vi "Intake.vi"() -> ()   [LabVIEW 2013]
uses:
  Globals/Homes.vi
  Globals/Useful Values.vi
  <vilib>/Rock Robotics/WPI/Joystick/WPI_JoystickGetSetRefNum.vi
  Robot Global Data.vi
  Globals/Auto.vi
  <vilib>/addons/control/pid/pid.llb/PID (DBL).vi
  <vilib>/addons/control/pid/NI_PID_pid.lvlib
panel:
  in  "x":dbl format="%#_13g"
  in  "PID gains Ultrasonic":T1={"proportional gain (Kc)"=12.0, "integral time (Ti, min)"=0.0, "derivative time (Td, min)"=0.0} {"derivative time (Td, min)" format="%.3f"; "integral time (Ti, min)" format="%.3f"; "proportional gain (Kc)" format="%.3f"}
  in  "Ultrasonic":dbl=0.6
  in  "Negate?":bool=TRUE
  out "Motor Output":dbl
  out "Intake Voltage":dbl=0.7652226560000001
  in  "PID gains":T1={"proportional gain (Kc)"=3.6, "integral time (Ti, min)"=0.0, "derivative time (Td, min)"=0.0} {"derivative time (Td, min)" format="%.3f"; "integral time (Ti, min)" format="%.3f"; "proportional gain (Kc)" format="%.3f"}
  out "Setpoint":dbl=0.75
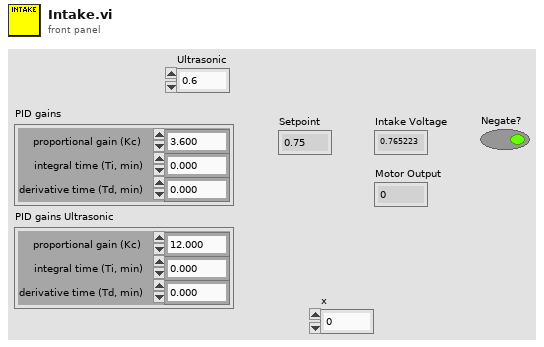
[diagram p1: front panel]
types:
  T1 = cluster{"proportional gain (Kc)":dbl, "integral time (Ti, min)":dbl, "derivative time (Td, min)":dbl}
  T2 = typedef "WPI_MotorControlDeviceRef.ctl" = cluster{"DeviceStatus":errorcluster, "Type":enum16{"PWM", "CAN"}, "PWM":cluster{"Digital Module":T3, "PWM Channel":T4, "DeadBand":T5}, "CAN":cluster{"Device Number":u8, "Control Mode":T6, "Semaphore":T7, "Max Vout":dbl}, "Invert":bool, "TransformRef":T8, "InvTransformRef":T8}
  T3 = typedef "FPGA_TypedefDigitalModule.ctl" = enum16{"Digital Module 1", "Digital Module 2"}
  T4 = typedef "FPGA_DIOPWMChannel.ctl" = enum8{"PWM 1", "PWM 2", "PWM 3", "PWM 4", "PWM 5", "PWM 6", "PWM 7", "PWM 8", "PWM 9", "PWM 10", "Invalid"}
  T5 = typedef "WPI_PWMDeadband.ctl" = cluster{"Name":string, "maxPositivePwm":i32, "minPositivePwm":i32, "centerPwm":i32, "maxNegativePwm":i32, "minNegativePwm":i32, "angularRange":u16}
  T6 = typedef "WPI_CANJaguar_ControlMode.ctl" = enum8{"Percent VBus", "Current", "Speed", "Position", "Voltage"}
  T7 = typedef "Semaphore RefNum" = refnum<k1>
  T8 = typedef "WPI_PWMTransform_ConPane.ctl" = refnum<vi>
  T9 = typedef "WPI_JoystickDevRef.ctl" = cluster{"Device":T10}
  T10 = typedef "WPI_JoystickDeviceEnum.ctl" = enum16{"USB 1", "USB 2", "USB 3", "USB 4", "Kinect 1", "Kinect 2"}
  T11 = typedef "WPI_AnalogChannelDevRef.ctl" = cluster{"DevStatus":errorcluster, "Analog Module":T12, "Analog Channel":T13}
  T12 = typedef "FPGA_TypedefAnalogModule.ctl" = enum16{"Analog Module 1", "Analog Module 2"}
  T13 = typedef "FPGA_AIChannel.ctl" = enum8{"AI 1", "AI 2", "AI 3", "AI 4", "AI 5", "AI 6", "AI 7", "AI 8", "Invalid"}
  T14 = typedef "WPI_DriverStationRobotMode2.ctl" = enum16{"Autonomous Disabled", "Autonomous Enabled", "Teleop Disabled", "Teleop Enabled", "Timeout", "Finish", "Test Disabled", "Test Enabled"}
  T15 = typedef "WPI_JoystickButtonState.ctl" = cluster{"Button 1":bool, "Button 2":bool, "Button 3":bool, "Button 4":bool, "Button 5":bool, "Button 6":bool, "Button 7":bool, "Button 8":bool, "Button 9":bool, "Button 10":bool, "Button 11":bool, "Button 12":bool}
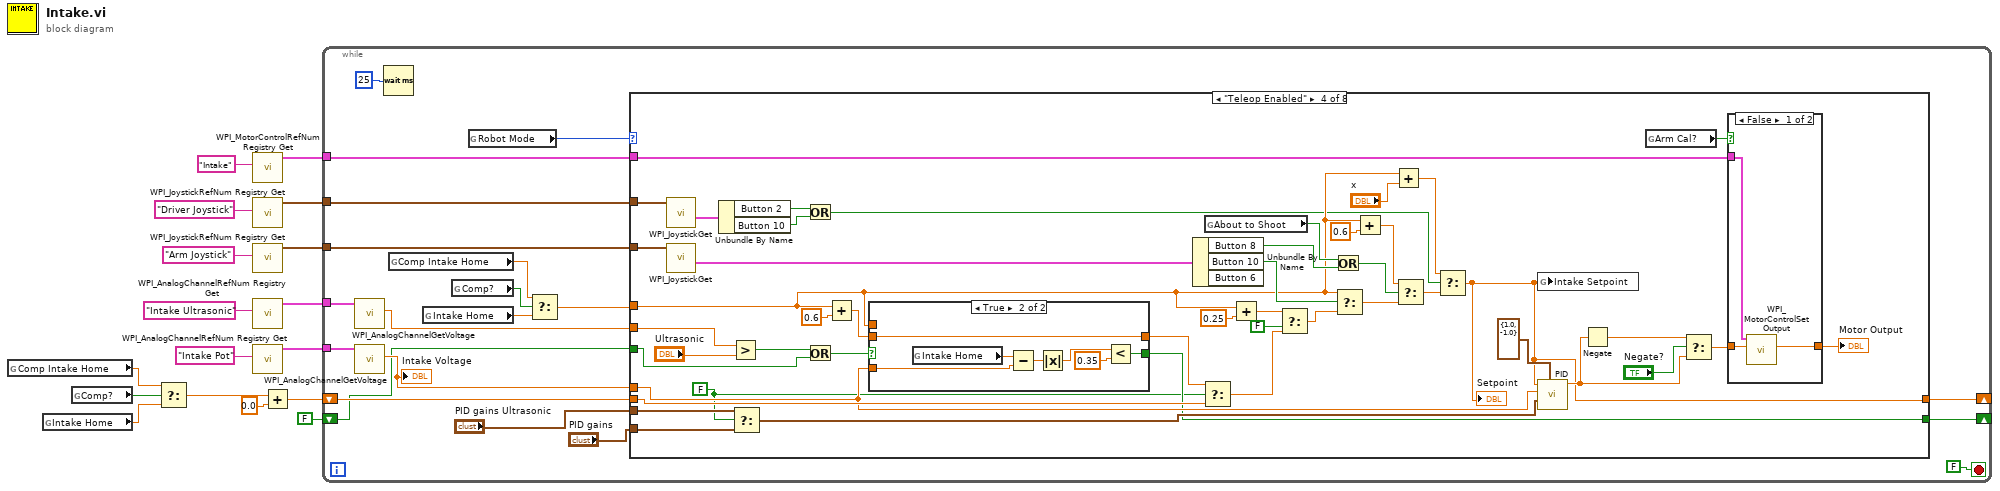
[diagram p0: block diagram]
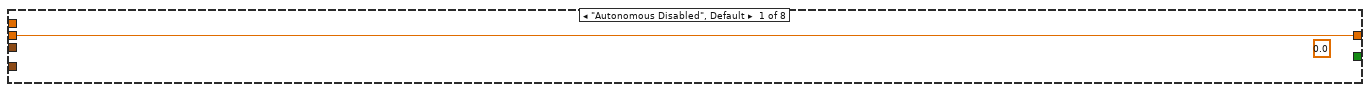
[diagram p2: hidden frame]
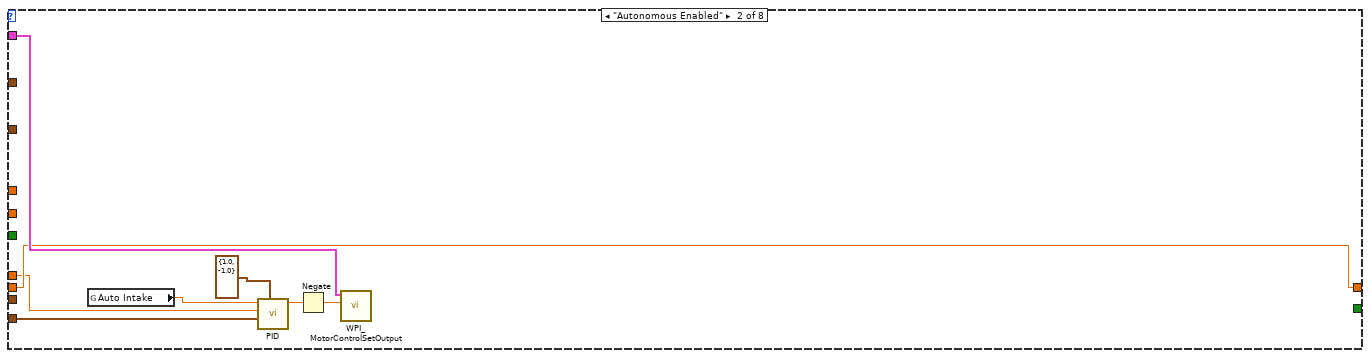
[diagram p3: hidden frame]
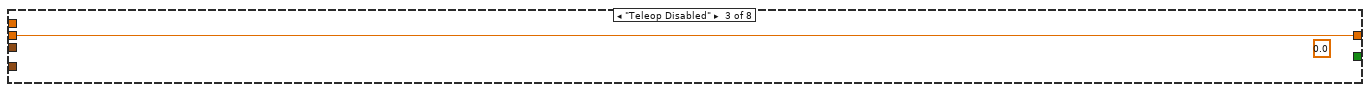
[diagram p4: hidden frame]
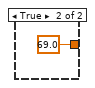
[diagram p5: hidden frame]
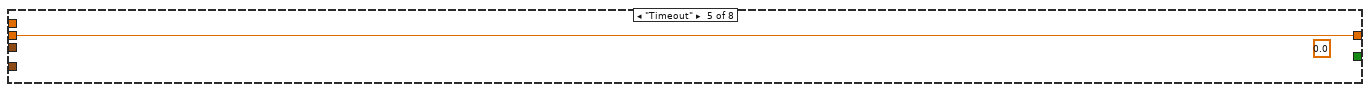
[diagram p7: hidden frame]
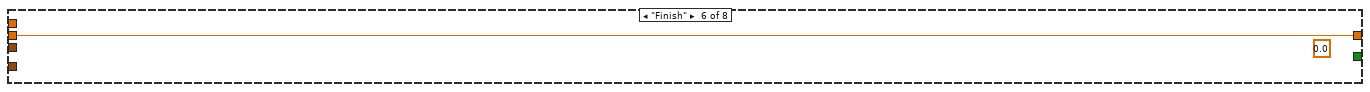
[diagram p8: hidden frame]
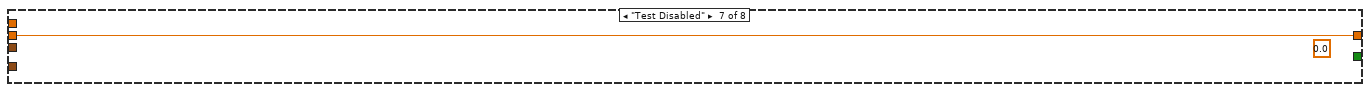
[diagram p9: hidden frame]
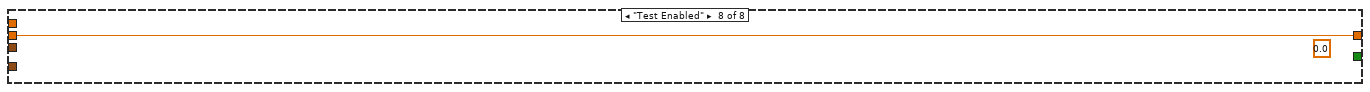
[diagram p10: hidden frame]
diagram:
  n1 = global read "Homes.vi" "Comp Intake Home"() -> (w9:dbl)
  n2 = global read "Homes.vi" "Intake Home"() -> (w10:dbl)
  n3 = global read "Useful Values.vi" "Comp?"() -> (w11:bool)
  n4 = Select(t=w9, s=w11, f=w10) -> (s? t:f=w8:dbl)
  n5 = call <vilib>:"WPI_MotorControlRefNum Registry Get.vi"("refnum name"="Intake") -> ("MotorControlDevRef"=w14:T2)  [unwired: 9 in, 1 out]
  n6 = call <vilib>:"WPI_JoystickRefNum Registry Get.vi"("refnum name"="Driver Joystick") -> ("JoystickDevRef"=w1:T9)  [unwired: 9 in, 1 out]
  n7 = call <vilib>:"WPI_JoystickRefNum Registry Get.vi"("refnum name"="Arm Joystick") -> ("JoystickDevRef"=w12:T9)  [unwired: 9 in, 1 out]
  n8 = call <vilib>:"WPI_AnalogChannelRefNum Registry Get.vi"("refnum name"="Intake Ultrasonic") -> ("AIDeviceRef"=w4:T11)  [unwired: 9 in, 1 out]
  n9 = call <vilib>:"WPI_AnalogChannelRefNum Registry Get.vi"("refnum name"="Intake Pot") -> ("AIDeviceRef"=w17:T11)  [unwired: 9 in, 1 out]
  n10 = Add(x=w8, y=0.0 ("x")) -> (x+y=w7:dbl)
  n11 = while {
    tunnel: w17 -> [w35]
    tunnel: w14 -> [w33]
    tunnel: w12 -> [w30]
    shift-right: [w28] -> _
    shift-left: w7 -> [w29]
    tunnel: w4 -> [w23]
    shift-right: [w20] -> _
    shift-left: FALSE -> [w19]
    tunnel: w1 -> [w18]
    stop <- FALSE stop-if-true
    n12 = call <vilib>:"WPI_AnalogChannelGetVoltage.vi"("AIDeviceRef"=w23) -> ("Voltage"=w22:dbl)  [unwired: 8 in, 2 out]
    n13 = call <vilib>:"WPI_AnalogChannelGetVoltage.vi"("AIDeviceRef"=w35) -> ("Voltage"=w32:dbl)  [unwired: 8 in, 2 out]
    "Intake Voltage" <- w32
    n14 = Wait (ms)(milliseconds to wait=u32 25) -> ()  [unwired: 1 out]
    n15 = global read "Homes.vi" "Comp Intake Home"() -> (w27:dbl)
    n16 = global read "Homes.vi" "Intake Home"() -> (w26:dbl)
    n17 = global read "Useful Values.vi" "Comp?"() -> (w25:bool)
    n18 = global read "Robot Global Data.vi" "Robot Mode"() -> (w34:T14)
    n19 = Select(t=w27, s=w25, f=w26) -> (s? t:f=w24:dbl)
    n20 = case shown="\"Teleop Enabled\"" w34 {
      tunnel: w33 -> [_ w44 _ w52 _ _ _ _]
      tunnel: w32 -> [_ w42 _ w70 _ _ _ _]
      tunnel: "PID gains" -> [_ w45 _ w73 _ _ _ _]
      tunnel: w30 -> [_ _ _ w93 _ _ _ _]
      tunnel: w29 -> [w38 w43 w47 w77 w108 w109 w110 w111]
      tunnel: w24 -> [_ _ _ w57 _ _ _ _]
      tunnel: [w38 w43 w47 w60 w108 w109 w110 w111] -> w28
      tunnel: w22 -> [_ _ _ w76 _ _ _ _]
      tunnel: "PID gains Ultrasonic" -> [_ _ _ w71 _ _ _ _]
      tunnel: [_ _ _ w69 _ _ _ _] -> w20
      tunnel: w19 -> [_ _ _ w67 _ _ _ _]
      tunnel: w18 -> [_ _ _ w63 _ _ _ _]
      frame "Autonomous Disabled", Default {
        (unwired) 0.0 ("Motor Output")
      }
      frame "Autonomous Enabled" {
        n21 = global read "Auto.vi" "Auto Intake"() -> (w41:dbl)
        n22 = call-poly <vilib>:"PID.vi"("output range"=cluster{"output high":dbl, "output low":dbl} {"output high"=1.0, "output low"=-1.0}, "PID gains"=w45, "process variable"=w42, "setpoint"=w41) -> ("output"=w40:dbl)  [unwired: 6 in, 1 out]
        n23 = Negate(x=w40) -> (-x=w39:dbl)
        n24 = call <vilib>:"WPI_MotorControlSetOutput.vi"("Output"=w39, "MotorControlDevRef"=w44) -> ()  [unwired: 7 in, 3 out]
      }
      frame "Teleop Disabled" {
        (unwired) 0.0 ("Motor Output")
      }
      frame "Teleop Enabled" {
        w53 = FALSE ("Button 4")
        n25 = call <vilib>:"WPI_JoystickGet.vi"("JoystickDevRef"=w63) -> ("Buttons"=w62:T15)  [unwired: 4 in, 2 out]
        n26 = call <vilib>:"WPI_JoystickGet.vi"("JoystickDevRef"=w93) -> ("Buttons"=w92:T15)  [unwired: 4 in, 2 out]
        n27 = Unbundle By Name(w62) -> ("Button 2"=w56:bool, "Button 10"=w55:bool)
        n28 = Greater?(x=w76, y="Ultrasonic") -> (0:w66:bool)
        n29 = Select(t=w71, s=w53, f=w73) -> (s? t:f=w72:T1)
        n30 = Or(x=w56, y=w55) -> (x .or. y?=w54:bool)
        n31 = Or(x=w66, y=w67) -> (x .or. y?=w68:bool)
        n32 = Add(x=w57, y=0.6) -> (x+y=w65:dbl)
        n33 = case shown="True" w68 {
          selector: w68 -> [w100 _]
          tunnel: w70 -> [_ w107]
          tunnel: [w100 w102] -> w69
          tunnel: w65 -> [_ w101]
          tunnel: w57 -> [w99 _]
          tunnel: [w99 w101] -> w64
          frame False {
          }
          frame True {
            n34 = global read "Homes.vi" "Intake Home"() -> (w106:dbl)
            n35 = Subtract(x=w106, y=w107) -> (x-y=w105:dbl)
            n36 = Absolute Value(x=w105) -> (abs(x)=w104:dbl)
            n37 = Less?(x=w104, y=0.35) -> (x < y?=w102:bool)
          }
        }
        n38 = Unbundle By Name(w92) -> ("Button 8"=w82:bool, "Button 10"=w91:bool)  [unwired: 1 out]
        n39 = Select(t=w64, s=w53, f=w77) -> (s? t:f=w78:dbl)
        n40 = global read "Useful Values.vi" "About to Shoot"() -> (w84:bool)
        n41 = Add(x=w57, y=0.25) -> (x+y=w80:dbl)
        n42 = Select(t=w80, s=FALSE, f=w78) -> (s? t:f=w81:dbl)
        n43 = Or(x=w84, y=w82) -> (x .or. y?=w83:bool)
        n44 = Select(t=w57, s=w91, f=w81) -> (s? t:f=w88:dbl)
        n45 = Add(x=w57, y=0.6 ("x")) -> (x+y=w90:dbl)
        n46 = Add(x=w57, y="x") -> (x+y=w58:dbl)
        n47 = Select(t=w90, s=w83, f=w88) -> (s? t:f=w61:dbl)
        n48 = Select(t=w58, s=w54, f=w61) -> (s? t:f=w60:dbl)
        "Setpoint" <- w60
        n49 = global write "Useful Values.vi" "Intake Setpoint"(w60) -> ()
        n50 = call-poly <vilib>:"PID.vi"("output range"=cluster{"output high":dbl, "output low":dbl} {"output high"=1.0, "output low"=-1.0}, "PID gains"=w72, "process variable"=w70, "setpoint"=w60) -> ("output"=w86:dbl)  [unwired: 6 in, 1 out]
        n51 = Negate(x=w86) -> (-x=w87:dbl)
        n52 = global read "Useful Values.vi" "Arm Cal?"() -> (w50:bool)
        n53 = Select(t=w87, s="Negate?", f=w86) -> (s? t:f=w51:dbl)
        n54 = case shown="False" w50 {
          tunnel: w52 -> [w97 _]
          tunnel: w51 -> [w96 _]
          tunnel: [w95 69.0 ("Motor Output")] -> w49
          frame False {
            n55 = call <vilib>:"WPI_MotorControlSetOutput.vi"("Output"=w96, "MotorControlDevRef"=w97) -> ("Motor Output"=w95:dbl)  [unwired: 7 in, 2 out]
          }
          frame True {
          }
        }
        "Motor Output" <- w49
      }
      frame "Timeout" {
        (unwired) 0.0 ("Motor Output")
      }
      frame "Finish" {
        (unwired) 0.0 ("Motor Output")
      }
      frame "Test Disabled" {
        (unwired) 0.0 ("Motor Output")
      }
      frame "Test Enabled" {
        (unwired) 0.0 ("Motor Output")
      }
    }
  }
